vi "C3--C4.vi"(7 "Scale":string, 8 "Command Info In":T2, 10 "C3 to C4":T1={"1a"=90.0, "1d"=45.31, "1s"=0.75}, 11 "Starting Position":T5) -> (0 "Command Info Out":T2)   [LabVIEW 2017]
uses:
  Support Code/Starting Position.ctl
  <vilib>/Rock Robotics/WPI/Framework/Command Status Info.ctl
  <vilib>/Rock Robotics/WPI/Framework/Completion Status.ctl
  <vilib>/Rock Robotics/WPI/Framework/Completion Notifier.ctl
  Block Clusters/C3--C4.ctl
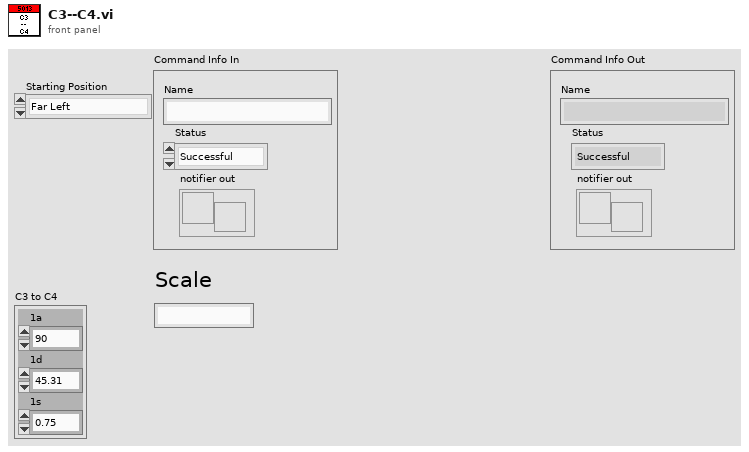
[diagram p1: front panel]
types:
  T1 = typedef "C3--C4.ctl" = cluster{"1a":dbl, "1d":dbl, "1s":dbl}
  T2 = typedef "Command Status Info.ctl" = cluster{"Name":string, "Status":T3, "notifier out":T4}
  T3 = typedef "Completion Status.ctl" = enum16{"Successful", "Aborted", "Incomplete"}
  T4 = typedef "Completion Notifier.ctl" = refnum<notifier>
  T5 = typedef "Starting Position.ctl" = enum16{"Far Left", "Middle", "Far Right"}
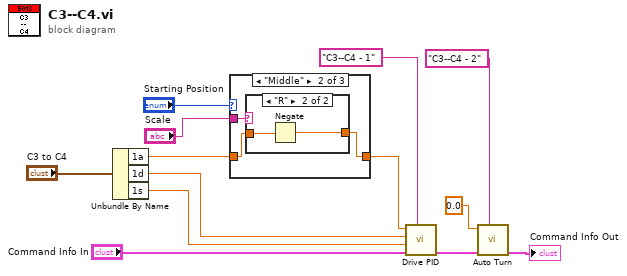
[diagram p0: block diagram]
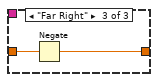
[diagram p4: hidden frame]
diagram:
  n1 = Unbundle By Name("C3 to C4") -> ("1a"=w6:dbl, "1d"=w5:dbl, "1s"=w4:dbl)
  n2 = case shown="\"Middle\"" "Starting Position" {
    tunnel: [w14 w16 w22] -> w11
    tunnel: w6 -> [w14 w17 w21]
    tunnel: "Scale" -> [_ w15 _]
    frame "Far Left", Default {
    }
    frame "Middle" {
      n3 = case shown="\"R\"" w15 {
        tunnel: w17 -> [w18 w20]
        tunnel: [w18 w19] -> w16
        frame "L", Default {
        }
        frame "R" {
          n4 = Negate(x=w20) -> (-x=w19:dbl)
        }
      }
    }
    frame "Far Right" {
      n5 = Negate(x=w21) -> (-x=w22:dbl)
    }
  }
  n6 = call "Drive PID.vi"("Description"="C3--C4 - 1", "Command Info In"="Command Info In", "Speed"=w4, "Distance"=w5, "Target Angle"=w11) -> ("Command Info Out"=w13:T2)  [unwired: 6 in]
  n7 = call "Auto Turn.vi"("Description"="C3--C4 - 2", "Command Info In"=w13, "Target Angle"=0.0) -> ("Command Info Out"=→"Command Info Out":T2)  [unwired: 8 in]
